vi "Array to String.vi"(7 "Strings? (F)":bool, 11 "JSON Strings":string[](array[string])) -> (3 "JSON Array String":string)   [LabVIEW 2020, in "JSON.lvlib"]
doc: "Converts an array of JSON strings to JSON array notation. Each input element will be separated by commas and the whole array will be enclosed with square braces \"[\" and \"]\".\n\nIf the JSON strings are intended to be treated as string values and not string representation of JSON objects, numerals, or other non-string values then ensure to set the <b>Strings?</b> input to True. This will wrap each element of the input strings in double-quotes and perform any necessary encoding."
uses:
  JSON.lvlib
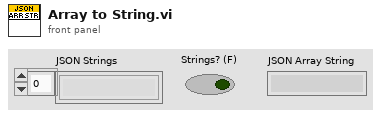
[diagram p1: front panel]
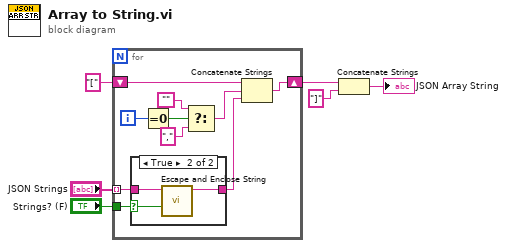
[diagram p0: block diagram]
diagram:
  n1 = for {
    shift-right: [w10] -> w5
    shift-left: "[" -> [w12]
    tunnel: "JSON Strings" -> [w8] mode=indexing
    tunnel: "Strings? (F)" -> [w9]
    i -> [w16]
    n2 = case shown="True" w9 {
      selector: w9 -> [_ w18]
      tunnel: w8 -> [w17 w20]
      tunnel: [w17 w19] -> w7
      frame False {
      }
      frame True {
        n3 = call "Escape and Enclose String.vi"("Force Enclose? (F)"=w18, "String"=w20) -> ("JSON String"=w19:string)  [unwired: 9 in]
      }
    }
    n4 = Equal To 0?(x=w16) -> (x = 0?=w15:bool)
    n5 = Select(t="", s=w15, f=",") -> (s? t:f=w11:string)
    n6 = Concatenate Strings(w12, w11, w7) -> (w10:string)
  }
  n7 = Concatenate Strings(w5, "]" ("string")) -> (→"JSON Array String":string)
